vi "GroveLedBlink.vi"() -> ()   [LabVIEW 2014]
doc: "GrovePi LED blink example for the Grove LED Socket (http://www.seeedstudio.com/wiki/Grove_-_LED_Socket_Kit)"
uses:
  GrovePi/Pin.ctl
  GrovePi/PinMode.ctl
  <vilib>/MakerHub/LINX/Public/Utilities/Open Local.vi
  LinxGrovePi/LinxGrovePi.lvclass
  <vilib>/MakerHub/LINX/LMH-LINX.lvlib
  GrovePi/GrovePi.lvclass
panel:
  in  "Pin":T1=4 items=["D2"=2, "D3"=3, "D4"=4, "D5"=5, "D6"=6, "D7"=7, "D8"=8, "D9"=9, "A0"=14, "A1"=15, "A2"=16, "A3"=17]
  out "Digital Status":bool
  in  "Stop Button":bool
  out "Error Out":errorcluster
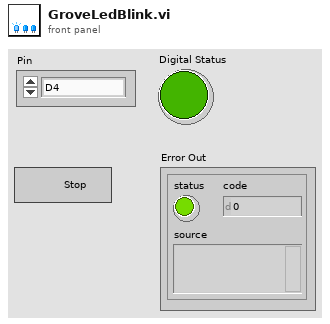
[diagram p1: front panel]
types:
  T1 = typedef "GrovePi.lvclass/Pin.ctl" = u8
  T2 = typedef "GrovePi.lvclass/PinMode.ctl" = u8
  T3 = typedef "LMH-LINX.lvlib/LINX Ref.ctl" = cluster{"IO":T4, "Interface":T5, "LINX Device Config":T6}
  T4 = typedef "LMH-LINX.lvlib/Platform.ctl" = enum16{"Remote", "Local"}
  T5 = typedef "LMH-LINX.lvlib/Interface.ctl" = enum16{"Serial", "TCP"}
  T6 = typedef "LMH-LINX.lvlib/Device.lvlib/LINX Device Config.ctl" = cluster{"Interface":T5, "COM Port":refnum<visa-resource-name>, "TCP Configuration":T7, "Device Family":u8, "Device ID":u8, "Device Name":string, "TCP Ref":refnum<k5>, "Channels":T8}
  T7 = typedef "LMH-LINX.lvlib/Device.lvlib/TCP Config.ctl" = cluster{"IP Address":string, "Port":u16}
  T8 = typedef "LMH-LINX.lvlib/Channels.ctl" = cluster{"DI":u8[], "DO":u8[], "AI":u8[], "AO":u8[], "PWM":u8[], "QE":u8[], "UART":u8[], "I2C 2":u8[], "SPI":u8[], "CAN":u8[], "Servo":u8[], "AI Ref (V)":dbl, "AI Resolution (Bits)":u8, "AO Ref (V)":dbl, "AO Resolution (Bits)":u8}
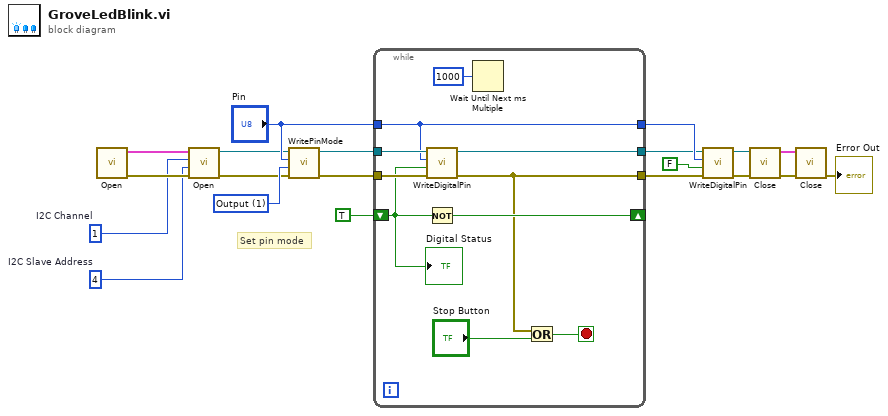
[diagram p0: block diagram]
diagram:
  w15 = T2 1 items=["Input", "Output"] ("Pin Mode")
  w16 = u8 4  # I2C Slave Address
  w17 = u8 1  # I2C Channel
  # "Set pin mode"
  n1 = call-poly <vilib>:"Open.vi"() -> ("Error Out"=w18:errorcluster, "LINX Resource"=w19:T3)  [unwired: 9 in, 1 out]
  n2 = call <vilib>:"Open.vi"("error in (no error)"=w18, "I2C Slave Address (4)"=w16, "I2C Channel (1)"=w17, "LINX Resource"=w19) -> ("error out"=w1:errorcluster, "LINX GrovePi out"=w2:refnum<class "LinxGrovePi.lvclass">)  [unwired: 6 in]
  n3 = call-dynamic "WritePinMode.vi"("error in (no error)"=w1, "Pin Mode"=w15, "Pin"="Pin", "GrovePi in"=w2) -> ("error out"=w13:errorcluster, "GrovePi out"=w14:refnum<class "LinxGrovePi.lvclass">)  [unwired: 6 in]
  n4 = while {
    tunnel: [w27] -> w9
    tunnel: [w24] -> w8
    tunnel: w14 -> [w29]
    tunnel: w13 -> [w28]
    shift-right: [w25] -> _
    shift-left: TRUE -> [w26]
    tunnel: "Pin" -> [w21]
    tunnel: [w21] -> w10
    stop <- w22 stop-if-true
    n5 = call-dynamic "WriteDigitalPin.vi"("error in (no error)"=w28, "Value"=w26, "Pin"=w21, "GrovePi in"=w29) -> ("error out"=w24:errorcluster, "GrovePi out"=w27:refnum<class "LinxGrovePi.lvclass">)  [unwired: 6 in]
    n6 = Not(x=w26) -> (.not. x?=w25:bool)
    n7 = Wait Until Next ms Multiple(millisecond multiple=u32 1000 ("milliseconds to wait")) -> ()  [unwired: 1 out]
    n8 = Or(x=w24, y="Stop Button") -> (x .or. y?=w22:bool)
    "Digital Status" <- w26
  }
  n9 = call-dynamic "WriteDigitalPin.vi"("error in (no error)"=w8, "Value"=FALSE, "Pin"=w10, "GrovePi in"=w9) -> ("error out"=w6:errorcluster, "GrovePi out"=w5:refnum<class "LinxGrovePi.lvclass">)  [unwired: 6 in]
  n10 = call <vilib>:"Close.vi"("error in (no error)"=w6, "LINX GrovePi in"=w5) -> ("error out"=w3:errorcluster, "LINX Resource"=w4:T3)  [unwired: 8 in]
  n11 = call <vilib>:"Close.vi"("Error In"=w3, "LINX Resource"=w4) -> ("Error Out"=→"Error Out":errorcluster)  [unwired: 9 in]
